vi "sendOutputs.vi"(8 "error in (no error)":errorcluster, 11 "ILC in":refnum<class "ILC.lvclass">) -> (0 "error out":errorcluster, 3 "ILC out":refnum<class "ILC.lvclass">)   [LabVIEW 2015, in "ILCCommon.lvlib" / "ILC.lvclass"]
uses:
  <userlib>/Common/ILC/ILC/ILC.lvclass
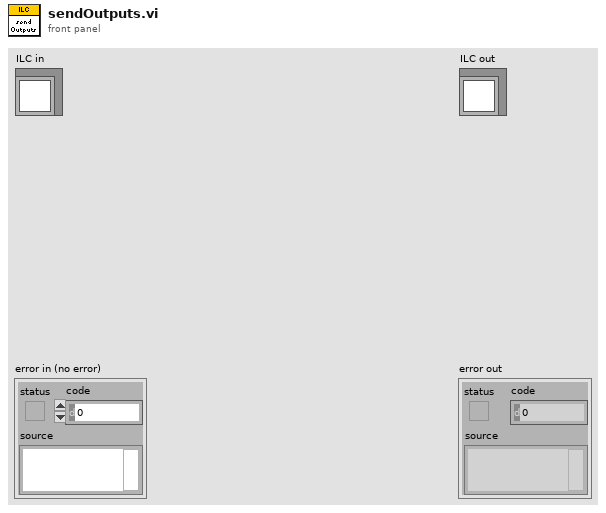
[diagram p1: front panel]
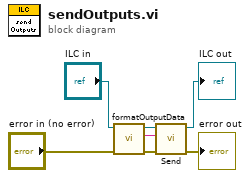
[diagram p0: block diagram]
diagram:
  n1 = call <userlib>:"formatOutputData.vi"("error in (no error)"="error in (no error)", "ILC in"="ILC in") -> ("error out"=w5:errorcluster, "formattedOutputData"=w4:string, "ILC out"=w3:refnum<class "ILC.lvclass">)  [unwired: 7 in]
  n2 = call-dynamic "Send.vi"("error in (no error)"=w5, "Message"=w4, "ILC in"=w3) -> ("error out"=→"error out":errorcluster, "ILC out"=→"ILC out":refnum<class "ILC.lvclass">)  [unwired: 7 in]
